vi "EatFeed.vi"(8 "error in (no error)":errorcluster, 11 "Snake in":refnum<class "Snake.lvclass">) -> (0 "error out":errorcluster, 3 "Snake out":refnum<class "Snake.lvclass">)   [LabVIEW 2018, in "Snake.lvclass"]
uses:
  Snake.lvclass
  Snake.lvclass/Snake.ctl
  Typedefs/CellType.ctl
  BodyCell/SnakeBodyCell.lvclass
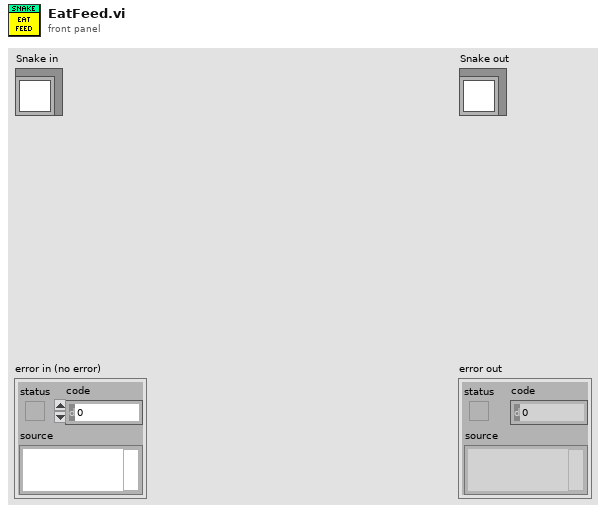
[diagram p1: front panel]
types:
  T1 = typedef "CellType.ctl" = enum16{"Head", "Tail", "Body"}
  T2 = typedef "Colors.ctl" = cluster{"HeadColor":u32, "BodyColor":u32, "TailColor":u32, "FeedColor":u32}
  T3 = typedef "DisplaySize.ctl" = cluster{"Rows":i32, "Cols":i32}
  T4 = typedef "UnitDirection.ctl" = enum16{"North", "East", "South", "West"}
  T5 = typedef "XYposition.ctl" = cluster{"Col.LocX":i32, "Row.LocY":i32}
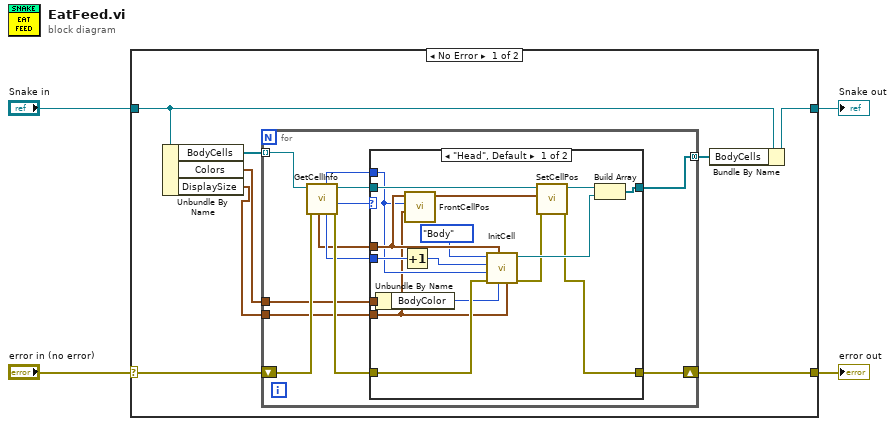
[diagram p0: block diagram]
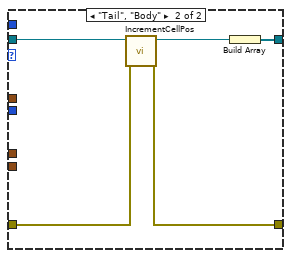
[diagram p2: hidden frame]
diagram:
  n1 = case shown="No Error" "error in (no error)" {
    selector: "error in (no error)" -> [w9 w47]
    tunnel: [w8 w47] -> w3
    tunnel: [w11 w46] -> w1
    tunnel: "Snake in" -> [w12 w46]
    frame No Error {
      n2 = Unbundle By Name(w12) -> ("BodyCells"=w10:refnum<class "SnakeBodyCell.lvclass">[], "Colors"=w6:T2, "DisplaySize"=w5:T3)
      n3 = for {
        tunnel: w10 -> [w24] mode=indexing
        tunnel: [w21] -> w7 mode=concatenating
        shift-right: [w18] -> w8
        shift-left: w9 -> [w23]
        tunnel: w6 -> [w14]
        tunnel: w5 -> [w13]
        n4 = call "GetCellInfo.vi"("error in (no error)"=w23, "SnakeBodyCell in"=w24) -> ("error out"=w19:errorcluster, "Cell"=w22:T1, "SnakeBodyCell out"=w20:refnum<class "SnakeBodyCell.lvclass">, "CellPosInBody"=w17:u16, "Direction"=w16:T4, "Position"=w15:T5)  [unwired: 2 in, 2 out]
        n5 = case shown="\"Head\", Default" w22 {
          tunnel: [w39 w41] -> w21
          tunnel: w20 -> [w38 w45]
          tunnel: w19 -> [w37 w43]
          tunnel: [w26 w42] -> w18
          tunnel: w17 -> [w36 _]
          tunnel: w16 -> [w28 _]
          tunnel: w15 -> [w32 _]
          tunnel: w14 -> [w34 _]
          tunnel: w13 -> [w25 _]
          frame "Head", Default {
            n6 = Unbundle By Name(w34) -> ("BodyColor"=w33:u32)
            n7 = Increment(x=w36) -> (x+1=w35:u16)
            n8 = call "FrontCellPos.vi"("DisplaySize"=w25, "Cell Direction"=w28, "Cell Pos"=w32) -> ("Front Cell Pos"=w29:T5)  [unwired: 8 in]
            n9 = call "InitCell.vi"("DisplaySize"=w25, "Color"=w33, "HeadPos"=w32, "error in (no error)"=w37, "Direction"=w28, "CellPosInBody"=w35, "Cell"=CellType."Body") -> ("error out"=w27:errorcluster, "SnakeBodyCell out"=w40:refnum<class "SnakeBodyCell.lvclass">)  [unwired: 3 in]
            n10 = call "SetCellPos.vi"("error in (no error)"=w27, "Position"=w29, "SnakeBodyCell in"=w38) -> ("error out"=w26:errorcluster, "SnakeBodyCell out"=w30:refnum<class "SnakeBodyCell.lvclass">)  [unwired: 7 in]
            n11 = Build Array(w30, w40) -> (w39:refnum<class "SnakeBodyCell.lvclass">[])
          }
          frame "Tail", "Body" {
            n12 = call "IncrementCellPos.vi"("error in (no error)"=w43, "SnakeBodyCell in"=w45) -> ("error out"=w42:errorcluster, "SnakeBodyCell out"=w44:refnum<class "SnakeBodyCell.lvclass">)  [unwired: 8 in]
            n13 = Build Array(w44) -> (w41:refnum<class "SnakeBodyCell.lvclass">[])
          }
        }
      }
      n14 = Bundle By Name(cluster=w12, "BodyCells"=w7) -> (w11:refnum<class "Snake.lvclass">)
    }
    frame Error {
    }
  }
  "error out" <- w3
  "Snake out" <- w1
